vi "SetFileAttributes.vi"() -> ()   [LabVIEW 2011]
uses:
  kernel32.dll
panel:
  out "error out":errorcluster
  in  "error in (no error)":errorcluster
  in  "FileName":string
  in  "File Attributes":cluster{bool, bool, bool, bool, bool, bool}
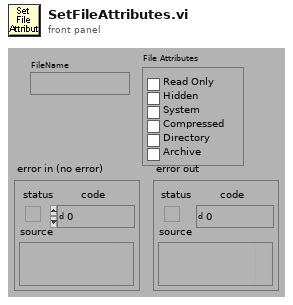
[diagram p1: front panel]
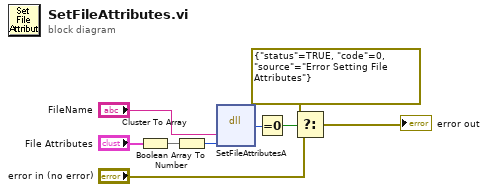
[diagram p0: block diagram]
diagram:
  n1 = Cluster To Array(cluster="File Attributes") -> (array=w8:bool[])
  n2 = Boolean Array To Number(Boolean array=w8) -> (number=w7:u32)
  n3 = dll-call lib="kernel32.dll" fn="SetFileAttributesA"("lpFileName"="FileName", "dwFileAttributes"=w7) -> (w5:u32)  [unwired: 5 in, 2 out]
  n4 = Equal To 0?(x=w5) -> (x = 0?=w4:bool)
  n5 = Select(t=errorcluster {"status"=TRUE, "code"=0, "source"="Error Setting File Attributes"}, s=w4, f="error in (no error)") -> (s? t:f=→"error out":errorcluster)
